vi "Average.vi"(0 "Data Avr in":T1, 1 "Size":i32, 5 "VALUE":dbl) -> (4 "Data Avr out":T1, 6 "AVR":dbl)   [LabVIEW 2019]
uses:
  Data Avr.ctl
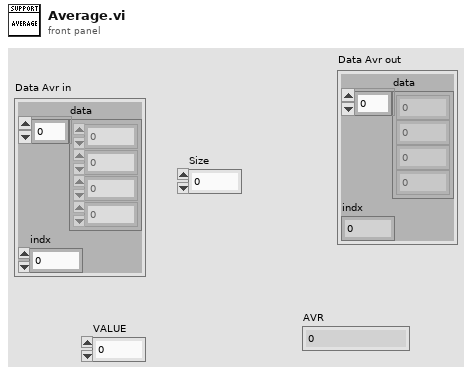
[diagram p1: front panel]
types:
  T1 = typedef "Data Avr.ctl" = cluster{"data":dbl[], "indx":i32}
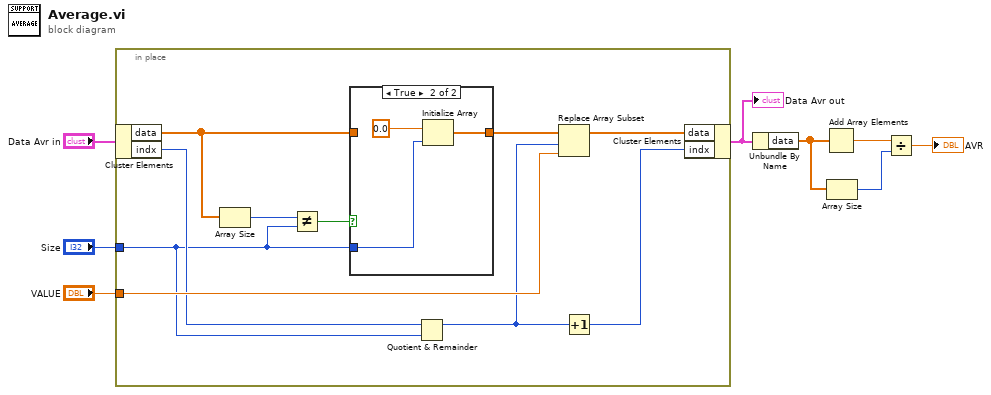
[diagram p0: block diagram]
diagram:
  n1 = in-place {
    in-place-border: "Size" -> [w11]
    in-place-border: "VALUE" -> [w13]
    n2 = in-place-cluster #1("Data Avr in") -> ("data"=w16:dbl[], "indx"=w12:i32)
    n3 = Array Size(array=w16) -> (size(s)=w18:i32)
    n4 = Not Equal?(x=w18, y=w11) -> (x != y?=w17:bool)
    n5 = case shown="True" w17 {
      tunnel: w16 -> [w19 _]
      tunnel: [w19 w20] -> w15
      tunnel: w11 -> [_ w21]
      frame False {
      }
      frame True {
        n6 = Initialize Array(0.0 ("element"), w21) -> (w20:dbl[])
      }
    }
    n7 = Quotient & Remainder(x=w12, y=w11) -> (x-y*floor(x/y)=w10:i32)  [unwired: 1 out]
    n8 = Replace Array Subset(array=w15, new element=w13, index=w10) -> (w14:dbl[])
    n9 = Increment(x=w10) -> (x+1=w9:i32)
    n10 = in-place-cluster #1("data"=w14, "indx"=w9) -> (w6:T1)
  }
  "Data Avr out" <- w6
  n11 = Unbundle By Name(w6) -> ("data"=w1:dbl[])
  n12 = Add Array Elements(numeric array=w1) -> (sum=w4:dbl)
  n13 = Array Size(array=w1) -> (size(s)=w5:i32)
  n14 = Divide(x=w4, y=w5) -> (x/y=→"AVR":dbl)
